vi "SystemToggle (1).vi"(8 "Enum In":T1=enum."Run", 11 "Activate/Deactivate System":bool) -> (0 "Enum Out":T1, 3 "PrePush Ready":bool)   [LabVIEW 2017]
doc: "Enables (or disables) subsystems in given, safe order: Disable Magnetic Brakes, Enable Suspension, Enable Levitation."
uses:
  SystemToggleEnum.ctl
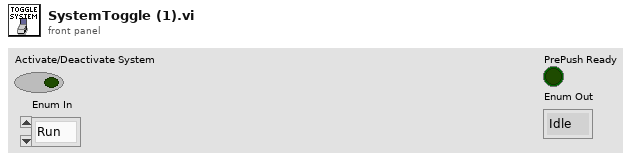
[diagram p1: front panel]
types:
  T1 = typedef "SystemToggleEnum.ctl" = enum16{"Idle", "MagBrake", "Suspension", "Levitation", "Run"}
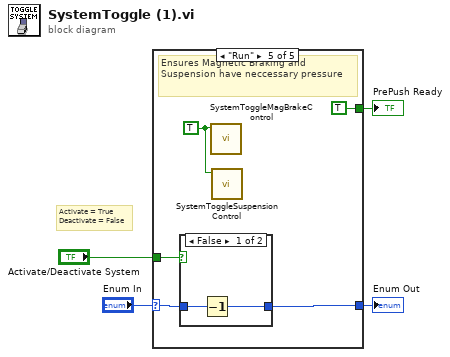
[diagram p0: block diagram]
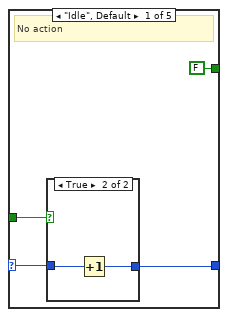
[diagram p2: hidden frame]
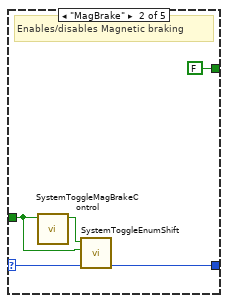
[diagram p4: hidden frame]
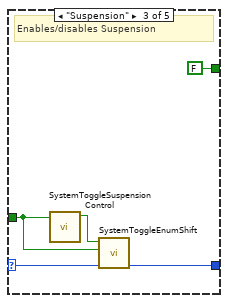
[diagram p5: hidden frame]
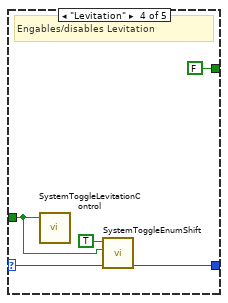
[diagram p6: hidden frame]
diagram:
  # "Activate = True\nDeactivate = False"
  n1 = case shown="\"Run\"" "Enum In" {
    selector: "Enum In" -> [w8 w15 w19 w25 w29]
    tunnel: "Activate/Deactivate System" -> [w7 w14 w20 w24 w30]
    tunnel: [w6 w16 w18 w26 w28] -> w1
    tunnel: [FALSE FALSE FALSE FALSE TRUE] -> w3
    frame "Idle", Default {
      # "No action"
      n2 = case shown="True" w7 {
        tunnel: w8 -> [w9 w11]
        tunnel: [w9 w10] -> w6
        frame False {
        }
        frame True {
          n3 = Increment(x=w11) -> (x+1=w10:T1)
        }
      }
    }
    frame "MagBrake" {
      # "Enables/disables Magnetic braking"
      n4 = call "SystemToggleMagBrakeControl.vi"("MagBrakeOn?"=w14) -> ("MagBrakeToggle Complete"=w13:bool)  [unwired: 10 in]
      n5 = call "SystemToggleEnumShift.vi"("Enum in"=w15, "On/Off"=w14, "Stage Complete"=w13) -> ("Enum"=w16:T1)  [unwired: 8 in]
    }
    frame "Suspension" {
      # "Enables/disables Suspension"
      n6 = call "SystemToggleSuspensionControl.vi"("SuspensionOn?"=w20) -> ("SuspensionToggle Complete"=w21:bool)  [unwired: 10 in]
      n7 = call "SystemToggleEnumShift.vi"("Enum in"=w19, "On/Off"=w20, "Stage Complete"=w21) -> ("Enum"=w18:T1)  [unwired: 8 in]
    }
    frame "Levitation" {
      # "Engables/disables Levitation"
      n8 = call "SystemToggleLevitationControl.vi"("LevitationControl"=w24) -> ()  [unwired: 11 in]
      n9 = call "SystemToggleEnumShift.vi"("Enum in"=w25, "On/Off"=w24, "Stage Complete"=TRUE) -> ("Enum"=w26:T1)  [unwired: 8 in]
    }
    frame "Run" {
      w31 = TRUE
      # "Ensures Magnetic Braking and Suspension have neccessary pressure"
      n10 = case shown="False" w30 {
        tunnel: w29 -> [w33 w34]
        tunnel: [w32 w34] -> w28
        frame False {
          n11 = Decrement(x=w33) -> (x-1=w32:T1)
        }
        frame True {
        }
      }
      n12 = call "SystemToggleMagBrakeControl.vi"("MagBrakeOn?"=w31) -> ()  [unwired: 10 in, 1 out]
      n13 = call "SystemToggleSuspensionControl.vi"("SuspensionOn?"=w31) -> ()  [unwired: 10 in, 1 out]
    }
  }
  "PrePush Ready" <- w3
  "Enum Out" <- w1
